vi "ASDA-A2_Control Mode Setting.vi"(8 "error in":errorcluster, 10 "Control Mode":enum32{"PT", "PR", "S", "T", "Sz", "Tz"}(ring), 11 "Buffer Data In":T1) -> (0 "error out":errorcluster, 3 "Buffer Data Out":T1)   [LabVIEW 2016]
uses:
  Data Def/ASDA-A2_Buffer Data.ctl
  Data Def/ASDA-A2_Read Register Data.ctl
  Data Def/ASDA-A2_Write Register Data.ctl
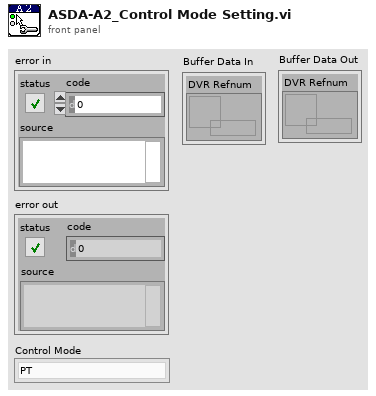
[diagram p1: front panel]
types:
  T1 = typedef "ASDA-A2_Buffer Data.ctl" = cluster{"DVR Refnum":refnum<data-value>}
  T2 = typedef "ASDA-A2_Read Register Data.ctl" = cluster{"Address":u16, "Count":u16, "Page":string, "Description":string}
  T3 = typedef "ASDA-A2_Write Register Data.ctl" = cluster{"Address":u16, "Max Value":u32, "Min Value":u32, "Value":u32, "Type":enum16{"16 Bits", "32 Bits"}, "Page":string, "Description":string}
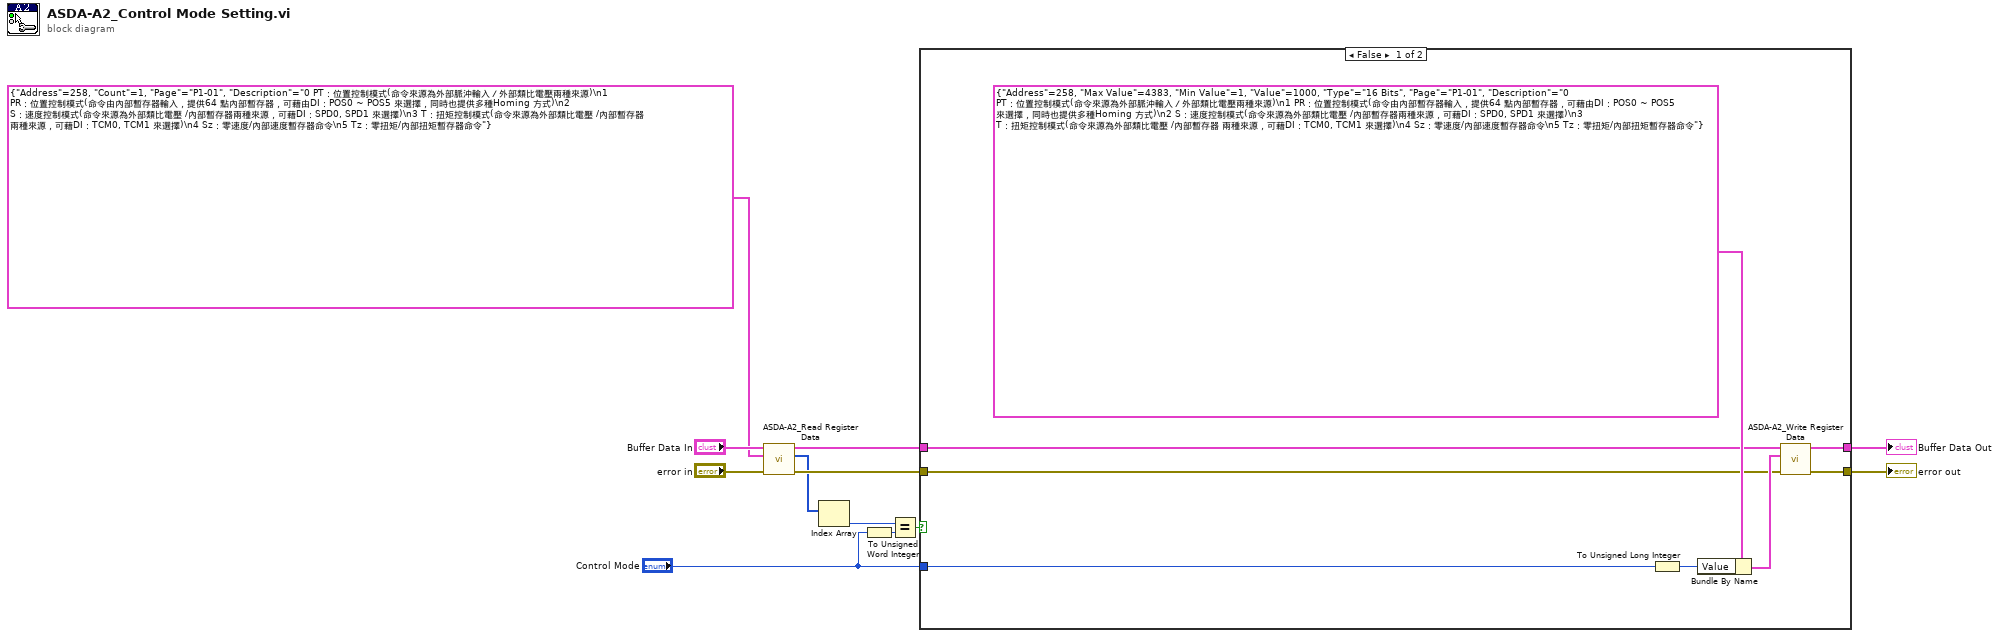
[diagram p0: block diagram]
diagram:
  n1 = call "ASDA-A2_Read Register Data.vi"("error in"="error in", "Read Register Data"=T2 {"Address"=258, "Count"=1, "Page"="P1-01", "Description"="0 PT：位置控制模式(命令來源為外部脈沖輸入／外部類比電壓兩種來源)\n1 PR：位置控制模式(命令由內部暫存器輸入，提供64 點內部暫存器，可藉由DI：POS0 ~ POS5 來選擇，同時也提供多種Homing 方式)\n2 S：速度控制模式(命令來源為外部類比電壓 /內部暫存器兩種來源，可藉DI：SPD0, SPD1 來選擇)\n3 T：扭矩控制模式(命令來源為外部類比電壓 /內部暫存器 兩種來源，可藉DI：TCM0, TCM1 來選擇)\n4 Sz：零速度/內部速度暫存器命令\n5 Tz：零扭矩/內部扭矩暫存器命令"}, "Buffer Data In"="Buffer Data In") -> ("error out"=w9:errorcluster, "Data"=w7:u16[], "Buffer Data Out"=w10:T1)  [unwired: 6 in]
  n2 = Index Array(array=w7) -> (element=w6:u16)  [unwired: 1 in]
  n3 = To Unsigned Word Integer(number="Control Mode") -> (unsigned 16bit integer=w5:u16)
  n4 = Equal?(x=w6, y=w5) -> (x = y?=w4:bool)
  n5 = case shown="False" w4 {
    tunnel: w10 -> [w17 w21]
    tunnel: w9 -> [w16 w22]
    tunnel: "Control Mode" -> [w15 _]
    tunnel: [w14 w21] -> w2
    tunnel: [w13 w22] -> w1
    frame False {
      n6 = To Unsigned Long Integer(number=w15) -> (unsigned 32bit integer=w19:u32)
      n7 = Bundle By Name(cluster=T3 {"Address"=258, "Max Value"=4383, "Min Value"=1, "Value"=1000, "Type"=enum."16 Bits", "Page"="P1-01", "Description"="0 PT：位置控制模式(命令來源為外部脈沖輸入／外部類比電壓兩種來源)\n1 PR：位置控制模式(命令由內部暫存器輸入，提供64 點內部暫存器，可藉由DI：POS0 ~ POS5 來選擇，同時也提供多種Homing 方式)\n2 S：速度控制模式(命令來源為外部類比電壓 /內部暫存器兩種來源，可藉DI：SPD0, SPD1 來選擇)\n3 T：扭矩控制模式(命令來源為外部類比電壓 /內部暫存器 兩種來源，可藉DI：TCM0, TCM1 來選擇)\n4 Sz：零速度/內部速度暫存器命令\n5 Tz：零扭矩/內部扭矩暫存器命令"} ("Write Register Data"), "Value"=w19) -> (w18:T3)
      n8 = call "ASDA-A2_Write Register Data.vi"("error in"=w16, "Write Register Data"=w18, "Buffer Data In"=w17) -> ("error out"=w13:errorcluster, "Buffer Data Out"=w14:T1)  [unwired: 7 in]
    }
    frame True {
    }
  }
  "error out" <- w1
  "Buffer Data Out" <- w2
